vi "IsEmpty.vi"(8 "error in (no error)":errorcluster, 11 "DataObject in":refnum<class "DataObject.lvclass">) -> (0 "error out":errorcluster, 3 "empty?":bool)   [LabVIEW 2015, in "UndoLibrary.lvlib" / "DataObject.lvclass"]
uses:
  DataObject.lvclass
  DataObject.lvclass/DataObject.ctl
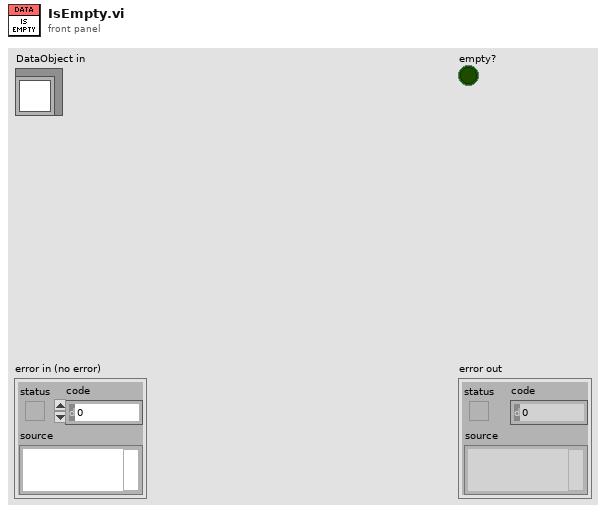
[diagram p1: front panel]
types:
  T1 = typedef "UndoLibrary.lvlib/DataObject.lvclass/cluster_Control Value.ctl" = cluster{"Index":i32, "Variant Data":variant}
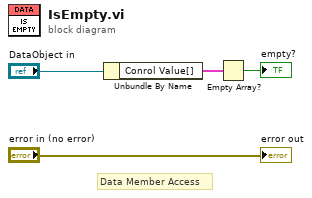
[diagram p0: block diagram]
diagram:
  # "Data Member Access"
  n1 = Unbundle By Name("DataObject in") -> ("Conrol Value[]"=w2:T1[])
  n2 = Empty Array?(array=w2) -> (empty?=→"empty?":bool)
  "error out" <- "error in (no error)"
